vi "createILC.vi"() -> (3 "ILC":refnum<class "ILC.lvclass">)   [LabVIEW 2015]
uses:
  <userlib>/Common/ILC/ILC/ILC.lvclass
  <userlib>/Common/SerialProtocols/SerialCommunicator/SerialCommunicator.lvclass
  <userlib>/Common/SerialProtocols/SerialProtocolFactory/SerialProtocolFactory/SerialProtocolFactory.lvclass
  Model/ILCTC/ILCTC.lvclass
  <userlib>/Common/SerialProtocols/SerialCommunicator/SerialCommunicator.lvclass/SerialCommunicator.ctl
  <userlib>/Common/ILC/ILC/ILC.lvclass/ILC.ctl
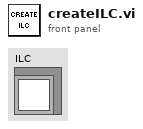
[diagram p1: front panel]
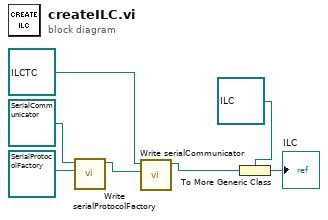
[diagram p0: block diagram]
diagram:
  n1 = call <userlib>:"Write serialProtocolFactory.vi"("serialProtocolFactory"=refnum<class "SerialProtocolFactory.lvclass"> refnum ("SerialProtocols.lvlib:SerialProtocolFactory.lvclass"), "SerialCommunicator in"=refnum<class "SerialCommunicator.lvclass"> refnum ("SerialProtocols.lvlib:SerialCommunicator.lvclass")) -> ("SerialCommunicator out"=w6:refnum<class "SerialCommunicator.lvclass">)  [unwired: 9 in]
  n2 = call <userlib>:"Write serialCommunicator.vi"("serialCommunicator"=w6, "ILC in"=refnum<class "ILCTC.lvclass"> refnum ("ILCTC.lvclass")) -> ("ILC out"=w2:refnum<class "ILCTC.lvclass">)  [unwired: 9 in]
  n3 = To More Generic Class(target class=refnum<class "ILC.lvclass"> refnum ("ILCCommon.lvlib:ILC.lvclass"), reference=w2) -> (generic class reference=→"ILC":refnum<class "ILC.lvclass">)
